vi "about_dialog.vi"() -> ()   [LabVIEW 2021, in "FirstXNode .xnode"]
uses:
  FirstXNode .xnode
panel:
  out "Survery Dialog":enum32{"Page 1", "Page 2"}(tab)
  in  "no":bool
  in  "yes":bool
  out "text":string="This is a simple XNode demo! \n \nHow do you like it?"
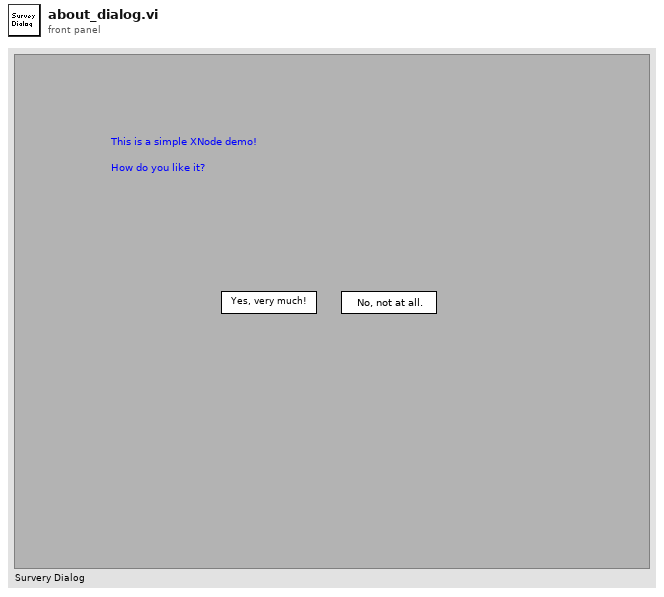
[diagram p1: front panel]
types:
  T1 = typedef "LVPoint32TypeDef.ctl" = cluster{"Horizontal":i32, "Vertical":i32}
  T2 = typedef "LVPositionTypeDef.ctl" = cluster{"Left":i32, "Top":i32}
  T3 = typedef "LVBoundsTypeDef.ctl" = cluster{"Width":u32, "Height":u32}
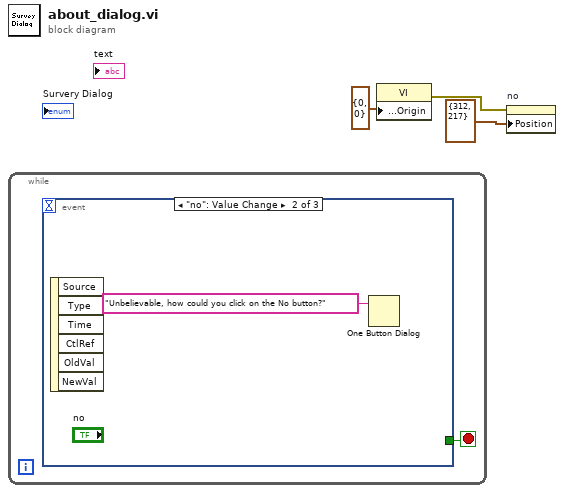
[diagram p0: block diagram]
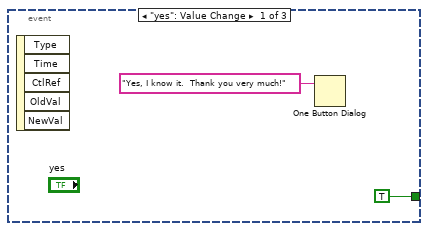
[diagram p2: hidden frame]
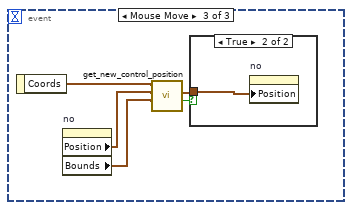
[diagram p3: hidden frame]
diagram:
  n1 = while {
    stop <- w4 stop-if-true
    n2 = event shown="[1] \"no\": Value Change" {
      selector: _ -> [_ _ _]
      dyn-events: _ -> [_ _ _]
      timeout: _ -> [_ _ _]
      tunnel: [TRUE _ _] -> w4
      event "yes": Value Change {
        n3 = event-data() -> ()  [unwired: 1 in, 5 out]
        n4 = One Button Dialog(message="Yes, I know it.  Thank you very much!") -> ()  [unwired: 1 in, 1 out]
      }
      event "no": Value Change {
        n5 = event-data() -> ()  [unwired: 1 in, 6 out]
        n6 = One Button Dialog(message="Unbelievable, how could you click on the No button?") -> ()  [unwired: 1 in, 1 out]
      }
      event Mouse Move {
        n7 = event-data() -> ("Coords"=w12:T1)  [unwired: 1 in]
        n8 = property on="no" class="Bool"() -> ("Position"=w11:T2, "Bounds"=w10:T3)  [unwired: 2 in, 2 out]
        n9 = call "get_new_control_position.vi"("control bounds"=w10, "control postion"=w11, "mouse position"=w12) -> ("in range"=w8:bool, "control postion new"=w9:cluster{"Left":i32, "Top":i32})  [unwired: 7 in]
        n10 = case shown="True" w8 {
          tunnel: w9 -> [_ w13]
          frame False {
          }
          frame True {
            n11 = property on="no" class="Bool"("Position"=w13) -> ()  [unwired: 2 in, 2 out]
          }
        }
      }
    }
  }
  n12 = property class="VI"("Front Panel Window:Origin"=cluster{"Horizontal":i16, "Vertical":i16} {"Horizontal"=0, "Vertical"=0}) -> (error out=w1:errorcluster)  [unwired: 2 in, 1 out]
  n13 = property on="no" class="Bool"(error in=w1, "Position"=cluster{"Left":i32, "Top":i32} {"Left"=312, "Top"=217}) -> ()  [unwired: 1 in, 2 out]
